vi "Obtain Queue.vi"(8 "Error In":errorcluster, 10 "Queue Name":string) -> (0 "Error Out":errorcluster, 3 "queue out":refnum<queue>)   [LabVIEW 2019, in "Queues.lvlib"]
uses:
  Queues.lvlib
  Message Cluster.ctl
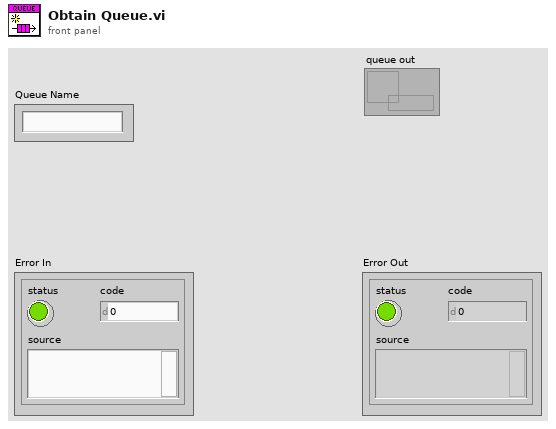
[diagram p1: front panel]
types:
  T1 = typedef "Queues.lvlib/Message Cluster.ctl" = cluster{"State":string, "Data":variant}
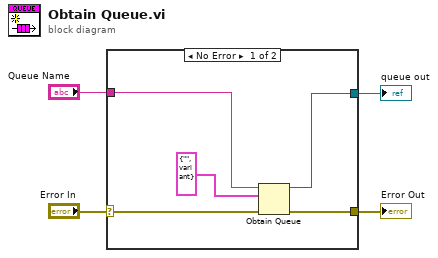
[diagram p0: block diagram]
diagram:
  n1 = case shown="No Error" "Error In" {
    selector: "Error In" -> [w9 w10]
    tunnel: [w8 w10] -> w3
    tunnel: "Queue Name" -> [w7 _]
    tunnel: [w5 _] -> w1
    frame No Error {
      n2 = Obtain Queue(name (unnamed)=w7, element data type=T1 {"State"="", "Data"=variant} ("Message"), error in (no error)=w9) -> (queue out=w5:refnum<queue>, error out=w8:errorcluster)  [unwired: 2 in, 1 out]
    }
    frame Error {
    }
  }
  "Error Out" <- w3
  "queue out" <- w1
